vi "Test Start.vi"(11 "Error in":errorcluster) -> (15 "Error out":errorcluster)   [LabVIEW 2020, in "StopWatchTests.lvlib"]
doc: "This VI is used for validating start button in stopwatch"
uses:
  StopWatchTests.lvlib
  <vilib>/SLL Drona/APIs/Stimulus/ControlValue/SetValueAuto.vi
  <vilib>/SLL Drona/APIs/Assert/AssertControlValue/Equal.vi
  <vilib>/SLL Drona/APIs/Get/GetControlValue/GetControlValueByPathString.vi
  <vilib>/SLL Drona/APIs/Stimulus/VI/CloseVI.vi
  <vilib>/addons/_JKI Toolkits/Caraya/classes/Test/Test.lvclass
  <vilib>/SLL Drona/Drona.lvlib
  <vilib>/SLL Drona/APIs/Stimulus/ControlValue/ControlValue.lvlib
  <vilib>/SLL Drona/APIs/Assert/AssertControlValue/AssertControlValue.lvlib
  <vilib>/SLL Drona/APIs/Get/GetControlValue/GetControlValue.lvlib
  <vilib>/SLL Drona/APIs/Stimulus/VI/VI.lvlib
panel:
  # "START TEST"
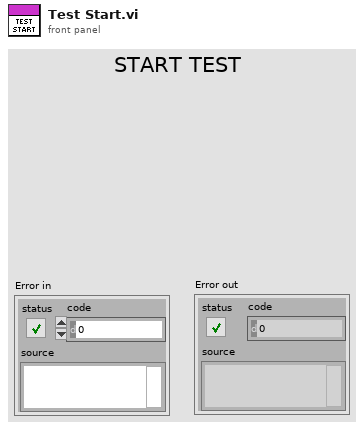
[diagram p1: front panel]
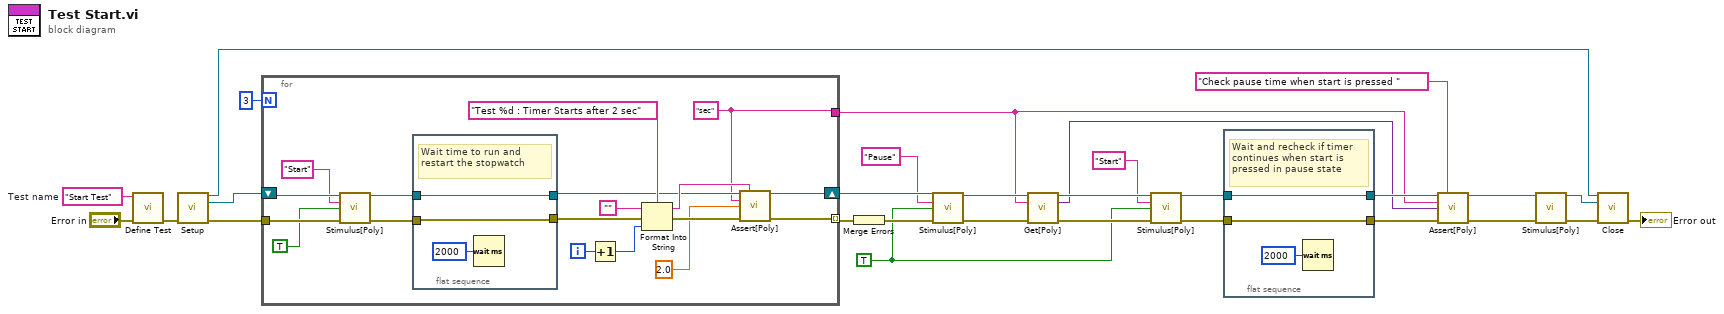
[diagram p0: block diagram]
diagram:
  w10 = TRUE
  w28 = "Start Test"  # Test name
  n1 = call <vilib>:"Define Test.vi"("error in (no error)"="Error in", "Label (VI Title)"=w28) -> ("error out"=w27:errorcluster)  [unwired: 9 in]
  n2 = call <vilib>:"Setup.vi"("error in"=w27) -> ("Application Ref"=w25:refnum<vi>, "VI Reference Out"=w20:refnum<vi>, "error out"=w21:errorcluster)  [unwired: 12 in]
  n3 = for {
    N: 3 -> [_]
    tunnel: w21 -> [w47]
    tunnel: [w32] -> w19 mode=indexing
    shift-right: [w31] -> w16
    shift-left: w20 -> [w46]
    tunnel: [w30] -> w1
    i -> [w37]
    w30 = "sec" ("Control Path")
    n4 = call-poly <vilib>:"Stimulus[Poly].vi"("VI Reference In"=w46, "Control Path"="Start", "Value (Signaling)"=TRUE, "error in"=w47) -> ("VI Reference Out"=w42:refnum<vi>, "error out"=w43:errorcluster)  [unwired: 10 in]
    n5 = flat-sequence {
      tunnel: w43 -> [w49]
      tunnel: [w49] -> w41
      tunnel: w42 -> [w48]
      tunnel: [w48] -> w34
      frame #0 {
        # "Wait time to run and restart the stopwatch"
        n6 = Wait (ms)(milliseconds to wait=u32 2000) -> ()  [unwired: 1 out]
      }
    }
    n7 = Increment(x=w37) -> (x+1=w36:i32)
    n8 = Format Into String(format string="Test %d : Timer Starts after 2 sec", initial string="", error in=w41, w36) -> (resulting string=w35:string, error out=w40:errorcluster)
    n9 = call-poly <vilib>:"Assert[Poly].vi"("VI Reference In"=w34, "Test Label"=w35, "Control Path"=w30, "Control Value"=2.0, "Error In"=w40) -> ("VI Reference Out"=w31:refnum<vi>, "Error Out"=w32:errorcluster)  [unwired: 9 in]
  }
  n10 = Merge Errors(w19) -> (w18:errorcluster)
  n11 = call-poly <vilib>:"Stimulus[Poly].vi"("VI Reference In"=w16, "Control Path"="Pause", "Value (Signaling)"=w10, "error in"=w18) -> ("VI Reference Out"=w13:refnum<vi>, "error out"=w17:errorcluster)  [unwired: 10 in]
  n12 = call-poly <vilib>:"Get[Poly].vi"("VI Reference In"=w13, "Control Path"=w1, "error in"=w17) -> ("VI Reference Out"=w12:refnum<vi>, "Value"=w4:variant, "error out"=w14:errorcluster)  [unwired: 10 in]
  n13 = call-poly <vilib>:"Stimulus[Poly].vi"("VI Reference In"=w12, "Control Path"="Start", "Value (Signaling)"=w10, "error in"=w14) -> ("VI Reference Out"=w8:refnum<vi>, "error out"=w9:errorcluster)  [unwired: 10 in]
  n14 = flat-sequence {
    tunnel: [w52] -> w7
    tunnel: w9 -> [w52]
    tunnel: w8 -> [w51]
    tunnel: [w51] -> w5
    frame #0 {
      # "Wait and recheck if timer continues when start is pressed in pause state"
      n15 = Wait (ms)(milliseconds to wait=u32 2000) -> ()  [unwired: 1 out]
    }
  }
  n16 = call-poly <vilib>:"Assert[Poly].vi"("VI Reference In"=w5, "Test Label"="Check pause time when start is pressed ", "Control Path"=w1, "Control Value"=w4, "Error In"=w7) -> ("VI Reference Out"=w2:refnum<vi>, "Error Out"=w6:errorcluster)  [unwired: 9 in]
  n17 = call-poly <vilib>:"Stimulus[Poly].vi"("VI Reference In"=w2, "error in"=w6) -> ("VI Reference Out"=w24:refnum<vi>, "error out"=w23:errorcluster)  [unwired: 12 in]
  n18 = call <vilib>:"Close.vi"("Application Ref"=w25, "VI Reference"=w24, "error in"=w23) -> ("error out"=→"Error out":errorcluster)  [unwired: 12 in]
